vi "Configure Time.vi"(0 "VISA resource name":refnum<visa-resource-name>, 5 "Hour (12)":i32=12 format="%02d", 7 "Minute (00)":i32 format="%02d", 11 "error IO":errorcluster, 12 "AM/PM (F:AM)":bool) -> (4 "VISA resource Out":refnum<visa-resource-name>, 15 "error Out":errorcluster)   [LabVIEW 2020, in "eec EST 300.lvlib"]
doc: "Sets the system time. Results will be returned as 2 digit integers. If 24 hour format is enabled the PM boolean should always be false."
uses:
  <instrlib>/eec EST 300/eec EST 300.lvlib
panel:
  # "PM\nAM"
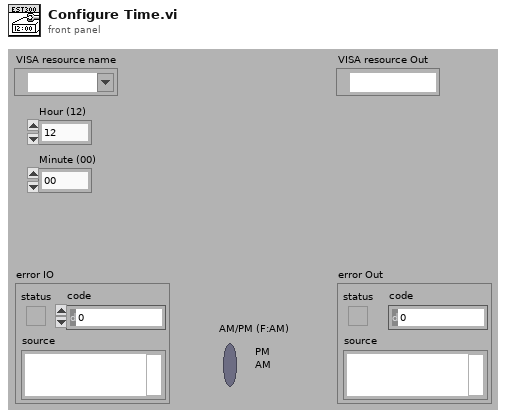
[diagram p1: front panel]
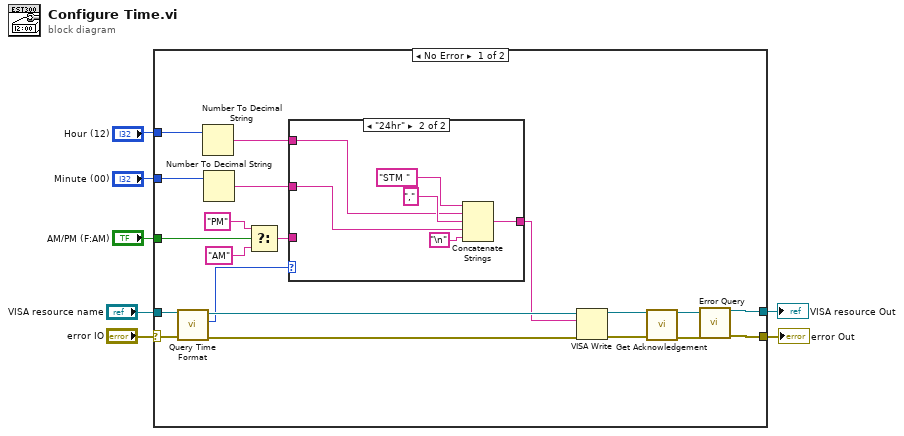
[diagram p0: block diagram]
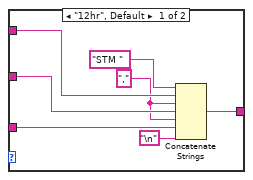
[diagram p2: hidden frame]
diagram:
  n1 = case shown="No Error" "error IO" {
    selector: "error IO" -> [w20 w42]
    tunnel: [w26 w42] -> w4
    tunnel: [w27 w41] -> w5
    tunnel: "VISA resource name" -> [w21 w41]
    tunnel: "Hour (12)" -> [w11 _]
    tunnel: "Minute (00)" -> [w10 _]
    tunnel: "AM/PM (F:AM)" -> [w9 _]
    frame No Error {
      n2 = call <instrlib>:"Query Time Format.vi"("error IO"=w20, "VISA resource name"=w21) -> ("error Out"=w19:errorcluster, "Time Format"=w8:enum16{"12hr", "24hr"}, "VISA resource Out"=w18:refnum<visa-resource-name>)  [unwired: 7 in]
      n3 = Number To Decimal String(number=w11) -> (decimal integer string=w15:string)  [unwired: 1 in]
      n4 = Number To Decimal String(number=w10) -> (decimal integer string=w14:string)  [unwired: 1 in]
      n5 = Select(t="PM" ("Command to Send (empty)"), s=w9, f="AM" ("Command to Send (empty)")) -> (s? t:f=w13:string)
      n6 = case shown="\"24hr\"" w8 {
        tunnel: [w34 w36] -> w12
        tunnel: w15 -> [w32 w38]
        tunnel: w14 -> [w31 w37]
        tunnel: w13 -> [w29 _]
        frame "12hr", Default {
          w30 = ","
          n7 = Concatenate Strings("STM " ("Command to Send (empty)"), w32, w30, w31, w30, w29, "\n") -> (w34:string)
        }
        frame "24hr" {
          n8 = Concatenate Strings("STM " ("Command to Send (empty)"), w38, ",", w37, "\n") -> (w36:string)
        }
      }
      n9 = VISA Write(VISA resource name=w18, write buffer=w12, error in (no error)=w19) -> (VISA resource name out=w23:refnum<visa-resource-name>, error out=w22:errorcluster)  [unwired: 1 out]
      n10 = call <instrlib>:"Get Acknowledgement.vi"("VISA resource name"=w23, "error in (no error)"=w22) -> ("VISA resource name out"=w25:refnum<visa-resource-name>, "error out"=w24:errorcluster)  [unwired: 12 in]
      n11 = call <instrlib>:"Error Query.vi"("VISA resource name"=w25, "error in (no error)"=w24) -> ("VISA resource name out"=w27:refnum<visa-resource-name>, "error out"=w26:errorcluster)  [unwired: 10 in, 2 out]
    }
    frame Error {
    }
  }
  "VISA resource Out" <- w5
  "error Out" <- w4
